vi "HFRR ADV v01.vi"() -> ()   [LabVIEW 2025] (continued)
          }
          frame #1 {
            n783 = local write "Tab Control 4"(T14."Air Step 3" ("Tab Control 4")) -> ()
          }
        }
      }
      event "Temperature Continue Step 3": Value Change {
        n784 = event-data() -> ()  [unwired: 1 in, 6 out]
        n785 = stacked-sequence {
          frame #0 {
            n786 = stacked-sequence {
              frame #0 {
                n787 = Wait (ms)(milliseconds to wait=u32 1500) -> ()  [unwired: 1 out]
              }
              frame #1 {
              }
              frame #2 {
              }
              frame #3 {
                # "CAL;A1;<true_T>"
                n788 = local write "Due Write"("CAL;A1;60" ("Command")) -> ()
              }
              frame #4 {
                n789 = Wait (ms)(milliseconds to wait=u32 1000) -> ()  [unwired: 1 out]
              }
              frame #5 {
                # "CAL;A1;<true_T>"
                n790 = local read "Sensor value"() -> (→"Sample 60deg temp":dbl)
                n791 = local write "Due Write"("CAL;A1;60" ("Command")) -> ()
              }
            }
          }
          frame #1 {
            w832 = 0.0
            w833 = 60.0
            n792 = local read "Sample 0deg temp"() -> (w843:dbl)
            n793 = local read "Sample 60deg temp"() -> (w842:dbl)
            n794 = Add(x=w833, y="Temperature diff") -> (x+y=w840:dbl)
            n795 = Subtract(x=w833, y="Temperature diff") -> (x-y=w839:dbl)
            n796 = Add(x=w832, y="Temperature diff") -> (x+y=w838:dbl)
            n797 = Subtract(x=w832, y="Temperature diff") -> (x-y=w837:dbl)
            n798 = In Range and Coerce(upper limit=w840, x=w842, lower limit=w839) -> (In Range?=w836:bool)  [unwired: 1 out]
            n799 = In Range and Coerce(upper limit=w838, x=w843, lower limit=w837) -> (In Range?=w835:bool)  [unwired: 1 out]
            n800 = And(x=w836, y=w835) -> (x .and. y?=w834:bool)
            n801 = case shown="True" w834 {
              frame False {
                n802 = property on="Accept & Save sample Temperature step 4" class="Bool (strict)"("DisabledEnum"=T20."Disabled" ("Disabled")) -> ()  [unwired: 2 in, 2 out]
                n803 = local write "Sample Temperature Calibration"(enum32{"True", "Fail"}."Fail" ("Sample Temperature Calibration  2")) -> ()
              }
              frame True {
                n804 = property on="Accept & Save sample Temperature step 4" class="Bool (strict)"("DisabledEnum"=T20."Enabled" ("Disabled")) -> ()  [unwired: 2 in, 2 out]
                n805 = local write "Sample Temperature Calibration"(enum32{"True", "Fail"}."True" ("Sample Temperature Calibration  2")) -> ()
              }
            }
          }
          frame #2 {
          }
          frame #3 {
          }
          frame #4 {
          }
          frame #5 {
          }
          frame #6 {
            # "CAL;END"
          }
          frame #7 {
          }
          frame #8 {
            # "CAL;END"
          }
          frame #9 {
            n806 = local write "Tab Control 4"(T14."Step 4" ("Tab Control 4")) -> ()
          }
        }
      }
      event "Accept & Save sample Temperature step 4": Value Change {
        n807 = event-data() -> ()  [unwired: 1 in, 6 out]
        n808 = stacked-sequence {
          frame #0 {
            n809 = local write "Due Write"("CAL;SAVE" ("Command")) -> ()
          }
          frame #1 {
            n810 = Wait (ms)(milliseconds to wait=u32 1000) -> ()  [unwired: 1 out]
          }
          frame #2 {
            n811 = local write "Due Write"("CAL;SAVE" ("Command")) -> ()
          }
          frame #3 {
            n812 = Wait (ms)(milliseconds to wait=u32 1000) -> ()  [unwired: 1 out]
          }
          frame #4 {
            n813 = local write "Due Write"("CAL;END" ("Command")) -> ()
          }
          frame #5 {
            n814 = Wait (ms)(milliseconds to wait=u32 1000) -> ()  [unwired: 1 out]
          }
          frame #6 {
            n815 = local write "Due Write"("CAL;END" ("Command")) -> ()
            n816 = local write "Temperature Selection"(T15."Default" ("Temperature Selection")) -> ()
            n817 = local write "Calibration Selection"(T10."Default" ("Calibration Selection")) -> ()
            n818 = local write "Tab Control 4"(T14."Main" ("Tab Control 4")) -> ()
            n819 = local write "Main Calibration Tab"(T9."Temperature" ("Main Calibration Tab")) -> ()
          }
          frame #7 {
            n820 = Get Date/Time In Seconds() -> (seconds since 1Jan1904=w862:timestamp)
            n821 = Format Into String(format string="%<%m/%d/%Y %I:%M:%S %p>T", w862) -> (resulting string=w860:string)  [unwired: 2 in, 1 out]
            n822 = local write "TEMPERATURE CALIBRATION"(w860) -> ()
          }
          frame #8 {
            n823 = local write "Save Button"(TRUE ("Save Button")) -> ()
            n824 = local write "Tab Control 4"(T14."Main" ("Tab Control 4")) -> ()
          }
        }
      }
      event "Accept & Save Air Temperature step 4": Value Change {
        n825 = event-data() -> ()  [unwired: 1 in, 6 out]
        n826 = stacked-sequence {
          frame #0 {
            n827 = local write "Due Write"("CAL;SAVE" ("Command")) -> ()
          }
          frame #1 {
            n828 = Wait (ms)(milliseconds to wait=u32 1000) -> ()  [unwired: 1 out]
          }
          frame #2 {
            n829 = local write "Due Write"("CAL;SAVE" ("Command")) -> ()
          }
          frame #3 {
            n830 = Wait (ms)(milliseconds to wait=u32 1000) -> ()  [unwired: 1 out]
          }
          frame #4 {
            n831 = local write "Due Write"("CAL;END" ("Command")) -> ()
          }
          frame #5 {
            n832 = Wait (ms)(milliseconds to wait=u32 1000) -> ()  [unwired: 1 out]
          }
          frame #6 {
            n833 = local write "Due Write"("CAL;END" ("Command")) -> ()
            n834 = local write "Tab Control 4"(T14."Main" ("Tab Control 4")) -> ()
            n835 = local write "Main Calibration Tab"(T9."Temperature" ("Main Calibration Tab")) -> ()
            n836 = local write "Temperature Selection"(T15."Default" ("Temperature Selection")) -> ()
            n837 = local write "Calibration Selection"(T10."Default" ("Calibration Selection")) -> ()
          }
          frame #7 {
            n838 = Get Date/Time In Seconds() -> (seconds since 1Jan1904=w878:timestamp)
            n839 = Format Into String(format string="%<%m/%d/%Y %I:%M:%S %p>T", w878) -> (resulting string=w877:string)  [unwired: 2 in, 1 out]
            n840 = local write "TEMPERATURE CALIBRATION"(w877) -> ()
          }
          frame #8 {
            n841 = local write "Tab Control 4"(T14."Main" ("Tab Control 4")) -> ()
            n842 = local write "Save Button"(TRUE ("Save Button")) -> ()
          }
        }
      }
      event "Temperature Continue Step 6": Value Change {
        n843 = event-data() -> ()  [unwired: 1 in, 6 out]
        n844 = stacked-sequence {
          frame #0 {
            n845 = stacked-sequence {
              frame #0 {
                n846 = Wait (ms)(milliseconds to wait=u32 1000) -> ()  [unwired: 1 out]
              }
              frame #1 {
              }
              frame #2 {
              }
              frame #3 {
                # "CAL;A1;<true_T>"
                n847 = local write "Due Write"("CAL;A1;60" ("Command")) -> ()
              }
              frame #4 {
                n848 = Wait (ms)(milliseconds to wait=u32 1000) -> ()  [unwired: 1 out]
              }
              frame #5 {
                # "CAL;A1;<true_T>"
                n849 = local write "Due Write"("CAL;A1;60" ("Command")) -> ()
              }
            }
          }
          frame #1 {
            n850 = local read "Sensor value"() -> (→"Air 60deg temp":dbl)
          }
          frame #2 {
          }
          frame #3 {
          }
          frame #4 {
          }
          frame #5 {
          }
          frame #6 {
            # "CAL;END"
          }
          frame #7 {
            w886 = 0.0 ("x")
            w887 = 60.0 ("x")
            n851 = local read "Temperature diff"() -> (w890:dbl)
            n852 = local read "Air 60deg temp"() -> (w889:dbl)
            n853 = local read "Air 0deg temp"() -> (w888:dbl)
            n854 = Add(x=w887, y=w890) -> (x+y=w897:dbl)
            n855 = Subtract(x=w887, y=w890) -> (x-y=w896:dbl)
            n856 = Add(x=w886, y=w890) -> (x+y=w895:dbl)
            n857 = Subtract(x=w886, y=w890) -> (x-y=w894:dbl)
            n858 = In Range and Coerce(upper limit=w897, x=w889, lower limit=w896) -> (In Range?=w893:bool)  [unwired: 1 out]
            n859 = In Range and Coerce(upper limit=w895, x=w888, lower limit=w894) -> (In Range?=w892:bool)  [unwired: 1 out]
            n860 = And(x=w893, y=w892) -> (x .and. y?=w891:bool)
            n861 = case shown="True" w891 {
              frame False {
                n862 = property on="Accept & Save Air Temperature step 4" class="Bool (strict)"("DisabledEnum"=T20."Disabled" ("Disabled")) -> ()  [unwired: 2 in, 2 out]
                n863 = local write "Air Temperature Calibration"(enum32{"True", "Fail"}."Fail" ("Sample Temperature Calibration  2")) -> ()
              }
              frame True {
                n864 = local write "Air Temperature Calibration"(enum32{"True", "Fail"}."True" ("Sample Temperature Calibration  2")) -> ()
                n865 = property on="Accept & Save Air Temperature step 4" class="Bool (strict)"("DisabledEnum"=T20."Enabled" ("Disabled")) -> ()  [unwired: 2 in, 2 out]
              }
            }
          }
          frame #8 {
            # "CAL;END"
          }
          frame #9 {
            n866 = local write "Tab Control 4"(T14."Air Step 4" ("Tab Control 4")) -> ()
          }
        }
      }
      event "Back Stroke step main temperature": Value Change {
        n867 = event-data() -> ()  [unwired: 1 in, 6 out]
        n868 = stacked-sequence {
          frame #0 {
            n869 = Wait (ms)(milliseconds to wait=u32 1000) -> ()  [unwired: 1 out]
          }
          frame #1 {
            # "CAL;END"
            n870 = local write "Due Write"("CAL;END" ("Command")) -> ()
          }
          frame #2 {
            n871 = Wait (ms)(milliseconds to wait=u32 1000) -> ()  [unwired: 1 out]
          }
          frame #3 {
            # "CAL;END"
            n872 = local write "Due Write"("CAL;END" ("Command")) -> ()
          }
          frame #4 {
            n873 = local write "Temperature Selection"(T15."Default" ("Temperature Selection")) -> ()
            n874 = local write "Calibration Selection"(T10."Default" ("Calibration Selection")) -> ()
            n875 = local write "Main Calibration Tab"(T9."Main" ("Main Calibration Tab")) -> ()
            n876 = local write "Tab Control 4"(T14."Main" ("Tab Control 4")) -> ()
          }
        }
      }
      event "TEMPERATURE STEP  Back 4", "TEMPERATURE STEP 1 Back 3", "TEMPERATURE STEP  Back 3", "TEMPERATURE STEP 1 Back 2", "Back Air TEMPERATURE Step 4", "Back SAMPLE TEMPERATURE Step 4": Value Change {
        # "Back Stroke step main temperature"
        n877 = event-data() -> ()  [unwired: 1 in, 6 out]
        n878 = stacked-sequence {
          frame #0 {
            n879 = Wait (ms)(milliseconds to wait=u32 1000) -> ()  [unwired: 1 out]
          }
          frame #1 {
            # "CAL;END"
            n880 = local write "Due Write"("CAL;END" ("Command")) -> ()
          }
          frame #2 {
            n881 = Wait (ms)(milliseconds to wait=u32 1000) -> ()  [unwired: 1 out]
          }
          frame #3 {
            # "CAL;END"
            n882 = local write "Due Write"("CAL;END" ("Command")) -> ()
          }
          frame #4 {
            # "TEMPERATURE STEP  Back 4"
            n883 = local write "Main Calibration Tab"(T9."Temperature" ("Main Calibration Tab")) -> ()
            n884 = local write "Temperature Selection"(T15."Default" ("Temperature Selection")) -> ()
            n885 = local write "Tab Control 4"(T14."Main" ("Tab Control 4")) -> ()
            n886 = local write "Calibration Selection"(T10."Default" ("Calibration Selection")) -> ()
          }
        }
      }
      event "FF BACK", "FF BACK 2", "FF BACK 3", "FF BACK 4", "FF BACK 5", "FF BACK 6": Value Change {
        n887 = event-data() -> ()  [unwired: 1 in, 6 out]
        n888 = stacked-sequence {
          frame #0 {
            n889 = Wait (ms)(milliseconds to wait=u32 1000) -> ()  [unwired: 1 out]
          }
          frame #1 {
            n890 = local write "Due Write"("VC;0") -> ()
          }
          frame #2 {
            n891 = Wait (ms)(milliseconds to wait=u32 1000) -> ()  [unwired: 1 out]
          }
          frame #3 {
            n892 = local write "Due Write"("VC;0") -> ()
          }
          frame #4 {
            w923 = FALSE
            n893 = local write "FF BACK 2"(w923) -> ()
            n894 = local write "FF BACK 3"(w923) -> ()
            n895 = local write "FF BACK 4"(w923) -> ()
            n896 = local write "FF BACK 5"(w923) -> ()
            n897 = local write "FF BACK 6"(w923) -> ()
            n898 = local write "FF BACK"(w923) -> ()
          }
          frame #5 {
            n899 = local write "Temperature Selection"(T15."Default" ("Temperature Selection")) -> ()
            n900 = local write "Calibration Selection"(T10."Default" ("Calibration Selection")) -> ()
            n901 = local write "Friction Force Tab"(T13."Page 1" ("Friction Force Tab")) -> ()
            n902 = local write "Main Calibration Tab"(T9."Main" ("Main Calibration Tab")) -> ()
            n903 = property on="Tab Control 6" class="TabCtl (strict)"("Visible"=FALSE) -> ()  [unwired: 2 in, 2 out]
            n904 = property on="Friction Force Calibration Result Tab" class="TabCtl (strict)"("Visible"=FALSE) -> ()  [unwired: 2 in, 2 out]
          }
        }
      }
      event "Accept & Save FF": Value Change {
        n905 = event-data() -> ()  [unwired: 1 in, 6 out]
        n906 = stacked-sequence {
          frame #0 {
            n907 = Wait (ms)(milliseconds to wait=u32 1000) -> ()  [unwired: 1 out]
          }
          frame #1 {
            n908 = local write "Due Write"("VC;0") -> ()
          }
          frame #2 {
            n909 = Wait (ms)(milliseconds to wait=u32 1000) -> ()  [unwired: 1 out]
          }
          frame #3 {
            n910 = local write "Due Write"("VC;0") -> ()
          }
          frame #4 {
            w934 = FALSE
            n911 = local write "FF BACK 2"(w934) -> ()
            n912 = local write "FF BACK 3"(w934) -> ()
            n913 = local write "FF BACK 4"(w934) -> ()
            n914 = local write "FF BACK 5"(w934) -> ()
            n915 = local write "FF BACK 6"(w934) -> ()
            n916 = local write "FF BACK"(w934) -> ()
          }
          frame #5 {
            n917 = Get Date/Time In Seconds() -> (seconds since 1Jan1904=w937:timestamp)
            n918 = Format Into String(format string="%<%m/%d/%Y %I:%M:%S %p>T", w937) -> (resulting string=w935:string)  [unwired: 2 in, 1 out]
            n919 = local write "FRICTION CALIBRATION"(w935) -> ()
          }
          frame #6 {
            n920 = local write "Temperature Selection"(T15."Default" ("Temperature Selection")) -> ()
            n921 = local write "Calibration Selection"(T10."Default" ("Calibration Selection")) -> ()
            n922 = local write "Friction Force Tab"(T13."Page 1" ("Friction Force Tab")) -> ()
            n923 = local write "Main Calibration Tab"(T9."Main" ("Main Calibration Tab")) -> ()
            n924 = local write "Save Button"(TRUE ("Save Button")) -> ()
            n925 = property on="Tab Control 6" class="TabCtl (strict)"("Visible"=FALSE) -> ()  [unwired: 2 in, 2 out]
            n926 = property on="Friction Force Calibration Result Tab" class="TabCtl (strict)"("Visible"=FALSE) -> ()  [unwired: 2 in, 2 out]
          }
        }
      }
      event "FF CONTINUE": Value Change {
        n927 = event-data() -> ()  [unwired: 1 in, 6 out]
        n928 = local write "FF CONTINUE"(FALSE ("FF CONTINUE")) -> ()
        n929 = local write "Friction Force Tab"(T13."Page 2" ("Friction Force Tab")) -> ()
      }
      event "FF CONTINUE 2": Value Change {
        n930 = event-data() -> ()  [unwired: 1 in, 6 out]
        n931 = local write "FF CONTINUE 2"(FALSE ("FF CONTINUE")) -> ()
        n932 = local write "Friction Force Tab"(T13."Page 3" ("Friction Force Tab")) -> ()
      }
      event "FF CONTINUE 3": Value Change {
        n933 = event-data() -> ()  [unwired: 1 in, 6 out]
        n934 = local write "FF CONTINUE 3"(FALSE ("FF CONTINUE")) -> ()
        n935 = local write "Friction Force Tab"(T13."Page 4" ("Friction Force Tab")) -> ()
      }
      event "FF CONTINUE 4": Value Change {
        n936 = event-data() -> ()  [unwired: 1 in, 6 out]
        n937 = local write "FF CONTINUE 4"(FALSE ("FF CONTINUE")) -> ()
        n938 = local write "Friction Force Tab"(T13."Page 5" ("Friction Force Tab")) -> ()
        n939 = property on="Friction Force Calibration Result Tab" class="TabCtl (strict)"("Visible"=FALSE) -> ()  [unwired: 2 in, 2 out]
      }
      event "FF CONTINUE 5": Value Change {
        n940 = event-data() -> ()  [unwired: 1 in, 6 out]
        n941 = local write "FF CONTINUE 5"(FALSE ("FF CONTINUE")) -> ()
        n942 = local write "Friction Force Tab"(T13."Page 6" ("Friction Force Tab")) -> ()
        n943 = property on="Friction Force Calibration Result Tab" class="TabCtl (strict)"("Visible"=FALSE) -> ()  [unwired: 2 in, 2 out]
        n944 = property on="Tab Control 6" class="TabCtl (strict)"("Visible"=FALSE) -> ()  [unwired: 2 in, 2 out]
      }
      event "Stroke Report Button": Value Change {
        n945 = event-data() -> ()  [unwired: 1 in, 6 out]
        n946 = local read "Point 5 - 1.0 mm"() -> (w959:bool)
        n947 = case shown="False" w959 {
          tunnel: [0.8 1.0] -> w958
          frame False {
          }
          frame True {
          }
        }
        n948 = local read "Machine Serial Number"() -> (w962:string)
        n949 = local read "USERNAME"() -> (w960:string)
        n950 = local write "Stroke Report Button"(FALSE ("Stroke Report Button")) -> ()
        n951 = call "Stroke Calibration Report.vi"("measured_value"=w958, "operator_name"=w960, "Instrument_serial Number"=w962) -> ()  [unwired: 7 in, 2 out]
      }
      event "Sample Report Button": Value Change {
        n952 = event-data() -> ()  [unwired: 1 in, 6 out]
        n953 = local read "Machine Serial Number"() -> (w968:string)
        n954 = local read "Sample 0deg temp"() -> (w965:dbl)
        n955 = local read "Sample 60deg temp"() -> (w966:dbl)
        n956 = local read "USERNAME"() -> (w967:string)
        n957 = call "Temperature Calibration Report.vi"("measured_60"=w966, "measured_zero"=w965, "operator_name"=w967, "Instrument_serial Number"=w968) -> ()  [unwired: 6 in, 2 out]
        n958 = local write "Sample Report Button"(FALSE ("Sample Report Button")) -> ()
      }
      event "Report Button FF": Value Change {
        n959 = event-data() -> ()  [unwired: 1 in, 6 out]
        n960 = local read "FF PASS"() -> (w973:bool)
        n961 = local read "Machine Serial Number"() -> (w976:string)
        n962 = Select(t="PASS", s=w973, f="FAIL") -> (s? t:f=w970:string)
        n963 = local read "USERNAME"() -> (w975:string)
        n964 = call "FF Calibration Report.vi"("pass_or_fail"=w970, "operator_name"=w975, "Instrument_serial Number"=w976) -> ()  [unwired: 7 in, 2 out]
        n965 = local write "Report Button FF"(FALSE ("Sample Report Button")) -> ()
      }
      event "Air Temperature Report Button": Value Change {
        n966 = event-data() -> ()  [unwired: 1 in, 6 out]
        n967 = local read "Machine Serial Number"() -> (w981:string)
        n968 = local read "Air 0deg temp"() -> (w978:dbl)
        n969 = local read "Air 60deg temp"() -> (w979:dbl)
        n970 = local read "USERNAME"() -> (w980:string)
        n971 = call "Air Temperature Calibration Report.vi"("measured_60"=w979, "measured_zero"=w978, "operator_name"=w980, "Instrument_serial Number"=w981) -> ()  [unwired: 6 in, 2 out]
        n972 = local write "Air Temperature Report Button"(FALSE ("Sample Report Button")) -> ()
      }
      event "Quit": Value Change {
        n973 = event-data() -> ()  [unwired: 1 in, 6 out]
      }
    }
    n974 = Wait (ms)(milliseconds to wait=u32 100) -> ()  [unwired: 1 out]
  }
  n975 = while {
    shift-right: [w984] -> _
    shift-left: "Enum - Selector" -> [w985]
    stop <- w986 stop-if-true
    # "Auto Start Logic Loop"
    n976 = case shown="\"close\"" w985 {
      tunnel: [w989 w995 w1023 w1058 w1088 Auto_Start_enum."Exit" ("Enum - Selector") Auto_Start_enum."Init" ("Enum - Selector")] -> w984
      frame "Init", Default {
        n977 = local read "Auto Start Test"() -> (w988:bool)
        n978 = Select(t=Auto_Start_enum."Humidity & Temperature On" ("Enum - Selector"), s=w988, f=Auto_Start_enum."Init") -> (s? t:f=w989:T17)
      }
      frame "Humidity & Temperature On" {
        n979 = stacked-sequence {
          tunnel: [_ _ _ _ _ _ Auto_Start_enum."Reach point" ("Enum - Selector")] -> w992
          frame #0 {
            w997 = T20."Disabled and Grayed Out" ("Disabled")
            w998 = TRUE ("Heater Button")
            n980 = property on="Humidity" class="Bool (strict)"("DisabledEnum"=w997) -> ()  [unwired: 2 in, 2 out]
            n981 = property on="Heater Button" class="Bool (strict)"("DisabledEnum"=w997) -> ()  [unwired: 2 in, 2 out]
            n982 = local write "Heater Button"(w998) -> ()
            n983 = local write "Humidity"(w998) -> ()
            n984 = property on="Heater Button" class="Bool (strict)"("Val(Sgnl)"=TRUE ("Value (Signaling)")) -> ()  [unwired: 2 in, 2 out]
          }
          frame #1 {
            n985 = Wait (ms)(milliseconds to wait=u32 3000) -> ()  [unwired: 1 out]
          }
          frame #2 {
            n986 = local read "Set Temp"() -> (w1004:dbl)
            n987 = Number To Fractional String(number=w1004, precision (6)=i16 2) -> (F-format string=w1001:string)  [unwired: 2 in]
            n988 = Concatenate Strings("ST;" ("Command"), w1001) -> (w1002:string)
            n989 = local write "Due Write"(w1002) -> ()
          }
          frame #3 {
            n990 = Wait (ms)(milliseconds to wait=u32 1500) -> ()  [unwired: 1 out]
          }
          frame #4 {
            (unwired) i16 2 ("precision (6)")
            n991 = local read "WriteHumidity"() -> (w1006:string[])
            n992 = local read "Set Rh"() -> (w1009:dbl)
            n993 = Number To Fractional String(number=w1009) -> (F-format string=w1010:string)  [unwired: 3 in]
            n994 = Concatenate Strings("M;" ("new element/subarray"), w1010) -> (w1011:string)
            n995 = Insert Into Array(array=w1006, new element=w1011) -> (w1007:string[])  [unwired: 1 in]
            n996 = local write "WriteHumidity"(w1007) -> ()
            n997 = local write "Due Write"("HE;1" ("Command")) -> ()
          }
          frame #5 {
            n998 = Wait (ms)(milliseconds to wait=u32 1500) -> ()  [unwired: 1 out]
          }
          frame #6 {
            w1014 = TRUE ("Reach point temp")
            n999 = local write "Reach point Humidity"(w1014) -> ()
            n1000 = local write "Reach point temp"(w1014) -> ()
          }
        }
        n1001 = local read "Auto Start Test"() -> (w994:bool)
        n1002 = Not(x=w994) -> (.not. x?=w993:bool)
        n1003 = Select(t=Auto_Start_enum."close", s=w993, f=w992) -> (s? t:f=w995:T17)
      }
      frame "Reach point" {
        w1024 = TRUE ("PAUSE")
        w1032 = 1.0 ("y")
        w1035 = 1.0 ("y")
        n1004 = local read "Set Temp"() -> (w1017:dbl)
        n1005 = local read "Set Humidity:"() -> (w1031:dbl)
        n1006 = local read "Humidity ( %RH )"() -> (w1036:dbl)
        n1007 = Add(x=w1017, y=w1035) -> (x+y=w1034:dbl)
        n1008 = Subtract(x=w1017, y=w1035) -> (x-y=w1033:dbl)
        n1009 = Add(x=w1031, y=w1032) -> (x+y=w1030:dbl)
        n1010 = Subtract(x=w1031, y=w1032) -> (x-y=w1029:dbl)
        n1011 = local read "TEMP"() -> (w1037:dbl)
        n1012 = In Range and Coerce(upper limit=w1030, x=w1036, lower limit=w1029) -> (In Range?=w1018:bool)  [unwired: 1 out]
        n1013 = In Range and Coerce(upper limit=w1034, x=w1037, lower limit=w1033) -> (In Range?=w1019:bool)  [unwired: 1 out]
        n1014 = disable-structure shown="Enabled" {
          disable-tunnel: w1018 -> [w1038 _]
          disable-tunnel: [w1038 TRUE] -> w1016
          frame Disabled {
            n1015 = case shown="True" w1038 {
              frame False {
              }
              frame True {
                n1016 = case shown="True" "Reach point Humidity" {
                  selector: "Reach point Humidity" -> [_ w1044]
                  frame False {
                  }
                  frame True {
                    n1017 = local read "EVENT LOG"() -> (w1041:string)
                    n1018 = Not(x=w1044) -> (.not. x?=w1043:bool)
                    n1019 = local write "Reach point Humidity"(w1043) -> ()
                    n1020 = call "Event Log.vi"("Content"="Target Humidity reached", "EVENT LOG"=w1041) -> ("EVENT LOG"=w1042:string)  [unwired: 8 in, 1 out]
                    n1021 = local write "EVENT LOG"(w1042) -> ()
                  }
                }
              }
            }
          }
          frame Enabled {
          }
        }
        n1022 = case shown="True" w1019 {
          frame False {
          }
          frame True {
            n1023 = case shown="True" "Reach point temp" {
              selector: "Reach point temp" -> [_ w1051]
              frame False {
              }
              frame True {
                n1024 = local read "EVENT LOG"() -> (w1048:string)
                n1025 = Not(x=w1051) -> (.not. x?=w1050:bool)
                n1026 = local write "Reach point temp"(w1050) -> ()
                n1027 = call "Event Log.vi"("Content"="Target Temperature reached", "EVENT LOG"=w1048) -> ("EVENT LOG"=w1049:string)  [unwired: 8 in, 1 out]
                n1028 = local write "EVENT LOG"(w1049) -> ()
              }
            }
          }
        }
        n1029 = local read "Auto Start Test"() -> (w1022:bool)
        n1030 = And(x=w1019, y=w1016) -> (x .and. y?=w1028:bool)
        n1031 = Select(t=Auto_Start_enum."Maintain Stage" ("Enum - Selector"), s=w1028, f=Auto_Start_enum."Reach point" ("Enum - Selector")) -> (s? t:f=w1025:T17)
        n1032 = Not(x=w1022) -> (.not. x?=w1021:bool)
        n1033 = Select(t=Auto_Start_enum."close", s=w1021, f=w1025) -> (s? t:f=w1023:T17)
        n1034 = call "ELAPSED TIMER VI.vi"("RESET"=w1024, "PAUSE"=w1024) -> ()  [unwired: 7 in, 3 out]
      }
      frame "Maintain Stage" {
        w1066 = 2.0 ("y")
        w1065 = 1.0 ("y")
        # "Humidity and temperature set point has stabilized."
        # "Humidity and  temperatures Set Point  have been reached"
        n1035 = local read "Set Temp"() -> (w1053:dbl)
        n1036 = local read "Set Humidity:"() -> (w1069:dbl)
        n1037 = local read "Humidity ( %RH )"() -> (w1072:dbl)
        n1038 = Add(x=w1053, y=w1065) -> (x+y=w1071:dbl)
        n1039 = Subtract(x=w1053, y=w1065) -> (x-y=w1070:dbl)
        n1040 = local read "TEMP"() -> (w1073:dbl)
        n1041 = Add(x=w1069, y=w1066) -> (x+y=w1068:dbl)
        n1042 = Subtract(x=w1069, y=w1066) -> (x-y=w1067:dbl)
        n1043 = In Range and Coerce(upper limit=w1071, x=w1073, lower limit=w1070) -> (In Range?=w1064:bool)  [unwired: 1 out]
        n1044 = In Range and Coerce(upper limit=w1068, x=w1072, lower limit=w1067) -> ()  [unwired: 2 out]
        n1045 = And(x=w1064, y=TRUE) -> (x .and. y?=w1063:bool)
        n1046 = Not(x=w1063) -> (.not. x?=w1062:bool)
        n1047 = call "ELAPSED TIMER VI.vi"("TARGET"=60.0, "RESET"=w1062, "PAUSE"=FALSE) -> ("ELAPSED INDICATION"=w1059:bool)  [unwired: 6 in, 2 out]
        n1048 = case shown="True" w1059 {
          tunnel: w1059 -> [_ w1076]
          tunnel: [Auto_Start_enum."Maintain Stage" ("Enum - Selector") w1075] -> w1057
          frame False {
          }
          frame True {
            n1049 = stacked-sequence {
              tunnel: w1076 -> [_ _ _ _ _]
              tunnel: [_ _ _ _ Auto_Start_enum."Start Stage" ("Enum - Selector")] -> w1075
              frame #0 {
                n1050 = local read "EVENT LOG"() -> (w1078:string)
                n1051 = call "Event Log.vi"("Content"="Temperature set point has stabilized.", "EVENT LOG"=w1078) -> ("EVENT LOG"=w1079:string)  [unwired: 8 in, 1 out]
                n1052 = local write "EVENT LOG"(w1079) -> ()
              }
              frame #1 {
                n1053 = Wait (ms)(milliseconds to wait=u32 100) -> ()  [unwired: 1 out]
              }
              frame #2 {
                n1054 = local read "EVENT LOG"() -> (w1083:string)
                n1055 = call "Event Log.vi"("Content"="Auto Test Started", "EVENT LOG"=w1083) -> ("EVENT LOG"=w1084:string)  [unwired: 8 in, 1 out]
                n1056 = local write "EVENT LOG"(w1084) -> ()
                n1057 = local write "FRICVALZ 4"(TRUE ("FRICVALZ 4")) -> ()
              }
              frame #3 {
                w1085 = TRUE ("RUN")
                n1058 = local write "RUN"(w1085) -> ()
                n1059 = property on="Auto Start Temp" class="Bool (strict)"("Val(Sgnl)"=w1085) -> ()  [unwired: 2 in, 2 out]
                "Auto Start Temp" <- w1085
              }
              frame #4 {
              }
            }
          }
        }
        n1060 = local read "Auto Start Test"() -> (w1056:bool)
        n1061 = Not(x=w1056) -> (.not. x?=w1055:bool)
        n1062 = Select(t=Auto_Start_enum."close", s=w1055, f=w1057) -> (s? t:f=w1058:T17)
      }
      frame "Start Stage" {
        w1087 = TRUE ("PAUSE")
        n1063 = local read "Auto Start Test"() -> (w1092:bool)
        n1064 = Not(x=w1092) -> (.not. x?=w1091:bool)
        n1065 = Select(t=Auto_Start_enum."close" ("Enum - Selector"), s=w1091, f=Auto_Start_enum."Start Stage" ("Enum - Selector")) -> (s? t:f=w1088:T17)
        n1066 = call "ELAPSED TIMER VI.vi"("RESET"=w1087, "PAUSE"=w1087) -> ()  [unwired: 7 in, 3 out]
      }
      frame "close" {
        w1095 = FALSE ("Heater Button")
        n1067 = local write "RUN"(w1095) -> ()
        n1068 = local write "Heater Button"(w1095) -> ()
        n1069 = local write "Humidity"(w1095) -> ()
        n1070 = local write "Auto Start Test"(w1095) -> ()
        n1071 = property on="Heater Button" class="Bool (strict)"("Val(Sgnl)"=FALSE ("Value (Signaling)")) -> ()  [unwired: 2 in, 2 out]
        n1072 = local write "Humidity 2"(TRUE ("Humidity")) -> ()
      }
      frame "Exit" {
      }
    }
    n1073 = Wait (ms)(milliseconds to wait=u32 100) -> ()  [unwired: 1 out]
    n1074 = local read "Quit"() -> (w986:bool)
  }
  n1075 = property on="Service Password Log" class="Str"("Visible"=w27) -> ()  [unwired: 2 in, 2 out]
  n1076 = property on="Password 3" class="Clust (strict)"("Visible"=w27) -> ()  [unwired: 2 in, 2 out]
  n1077 = while {
    stop <- w1124 stop-if-true
    w1107 = errorcluster {"status"=FALSE, "code"=0, "source"=""} ("error in (no error) 3")
    # "this loop is for manual report generation"
    n1078 = local read "Confirm Measrurement"() -> (w1106:bool)
    n1079 = case shown="True" w1106 {
      selector: w1106 -> [_ w1214]
      tunnel: errorcluster {"status"=FALSE, "code"=0, "source"=""} ("error in (no error) 3") -> [_ w1215]
      tunnel: [_ w1213] -> _
      frame False {
      }
      frame True {
        n1080 = stacked-sequence {
          tunnel: w1215 -> [_ w1248 _]
          tunnel: w1214 -> [_ _ w1355]
          tunnel: [_ w1236 _] -> w1213
          frame #0 {
            n1081 = String To Path(string="C:\\LAB-IQ\\Image Calibrate v01.dcf") -> (path=w1218:path)
            n1082 = Open/Create/Replace File ("Open File")(file path (use dialog)=w1218) -> (refnum out=w1219:refnum<file>)  [unwired: 5 in, 2 out]
            n1083 = for {
              N: 4 -> [_]
              tunnel: w1219 -> [w1225]
              i -> [w1221]
              n1084 = Read from Text File ("Read File")(file (use dialog)=w1225) -> (text=w1226:string)  [unwired: 3 in, 3 out]
              n1085 = String Subset(string=w1226, offset (0)=6, length (rest)=10 ("length (rest)")) -> (substring=w1222:string)
              n1086 = Fract/Exp String To Number(string=w1222) -> (number=w1220:dbl)  [unwired: 3 in, 1 out]
              n1087 = case shown="3" w1221 {
                tunnel: w1220 -> [w1227 w1228 _ w1229 _]
                frame 0 {
                  n1088 = local write "5x Gain"(w1227) -> ()
                }
                frame 1 {
                  n1089 = local write "10x Gain"(w1228) -> ()
                }
                frame 2 {
                }
                frame 3 {
                  n1090 = local write "100x gain"(w1229) -> ()
                }
                frame 4, Default {
                }
              }
            }
          }
          frame #1 {
            n1091 = local read "TEST STANDARD"() -> (w1231:T5)
            n1092 = case shown="\"ISO 12156\"" w1231 {
              tunnel: ["ASTM D6079" "ISO 12156"] -> w1230
              frame "ASTM D6079", Default {
              }
              frame "ISO 12156" {
              }
            }
            n1093 = call "IMAGE ANALYSIS.vi"("Enum"=POST_ANALYSIS_ENUM."GET MEASUREMENTS", "error in"=w1248) -> ("error out"=w1255:errorcluster)  [unwired: 8 in, 1 out]
            n1094 = local read "Magnification :"() -> (w1241:string)
            n1095 = call "Stall Data Flow.vim"("value in"=w1255, "milliseconds to wait"=u32 1000) -> ("value out"=w1254:errorcluster)  [unwired: 1 out]
            n1096 = local read "Test File List :"() -> (w1252:string)
            n1097 = case shown="\"10x\"" w1241 {
              tunnel: [w1291 w1292] -> w1239
              frame "5x", Default {
                n1098 = local read "5x Gain"() -> (w1291:dbl)
              }
              frame "10x" {
                # "5x"
                n1099 = local read "10x Gain"() -> (w1292:dbl)
              }
            }
            n1100 = call "IMAGE ANALYSIS.vi"("Enum"=POST_ANALYSIS_ENUM."READ", "error in"=w1254) -> ("error out"=w1251:errorcluster, "data out"=w1242:string)  [unwired: 8 in]
            n1101 = Match Pattern(string=w1242, regular expression="\"type\": ") -> (after substring=w1246:string)  [unwired: 1 in, 3 out]
            n1102 = call "IMAGE PATH CREATION PY.vi"("error in (no error)"=w1251, "File Name :"=w1252) -> ("error out"=w1250:errorcluster, "File Path"=w1238:path, "File Path String:"=w1233:string)  [unwired: 7 in]
            n1103 = Match Pattern(string=w1246, regular expression=",") -> (before substring=w1232:string)  [unwired: 1 in, 3 out]
            n1104 = local read "Calibration Tab"() -> (w1235:enum32{"Measrument", "Calibrate"})
            n1105 = call "Stall Data Flow.vim"("value in"=w1250, "milliseconds to wait"=u32 250) -> ("value out"=w1234:errorcluster)  [unwired: 1 out]
            n1106 = Equal?(x=w1232, y="\"rectangle\"") -> (x = y?=w1243:bool)
            n1107 = case shown="False" w1243 {
              tunnel: w1242 -> [w1297 w1352]
              tunnel: w1239 -> [_ w1343]
              tunnel: cluster{"major":dbl, "minor":dbl, "average":dbl} {"major"=0.0, "minor"=0.0, "average"=0.0} -> [w1295 w1339]
              tunnel: [w1294 w1336] -> w1237
              tunnel: w1232 -> [w1296 _]
              tunnel: w1239 -> [w1293 _]
              frame False {
                n1108 = Equal?(x=w1296, y="\"line\"") -> (x = y?=w1298:bool)
                n1109 = case shown="True" w1298 {
                  tunnel: w1297 -> [_ w1313]
                  tunnel: w1295 -> [w1300 w1312]
                  tunnel: [w1300 w1310] -> w1294
                  tunnel: w1293 -> [_ w1309]
                  frame False {
                  }
                  frame True {
                    w1308 = 0.0 ("Major Axis")
                    n1110 = Match Pattern(string=w1313, regular expression="\"length_px\":") -> (after substring=w1311:string)  [unwired: 1 in, 3 out]
                    n1111 = property on="Major Axis" class="DigNum (strict)"("Caption.Text"="") -> ()  [unwired: 2 in, 2 out]
                    n1112 = property on="Minor Axis" class="DigNum (strict)"("Caption.Text"="") -> ()  [unwired: 2 in, 2 out]
                    n1113 = property on="Average" class="DigNum (strict)"("Caption.Text"="Line") -> ()  [unwired: 2 in, 2 out]
                    n1114 = Fract/Exp String To Number(string=w1311, default (0 dbl)=0.0 ("default (0 DBL)")) -> (number=w1307:dbl)  [unwired: 2 in, 1 out]
                    "Pixel Value" <- w1307
                    n1115 = Multiply(x=w1307, y=w1309) -> (x*y=w1320:dbl)
                    n1116 = Multiply(x=w1320, y=1000.0) -> (x*y=w1303:dbl)
                    n1117 = Divide(x=w1303, y=1000.0) -> (x/y=w1306:dbl)
                    n1118 = local write "Measurment (mm)"(w1306) -> ()
                    n1119 = Bundle By Name(cluster=w1312, "average"=w1303) -> (w1310:cluster{"major":dbl, "minor":dbl, "average":dbl})
                    n1120 = Number To Fractional String(number=w1303, precision (6)=i16 1) -> (F-format string=w1302:string)  [unwired: 2 in]
                    n1121 = local write "Minor Axis"(w1308) -> ()
                    n1122 = local write "Major Axis"(w1308) -> ()
                    n1123 = Fract/Exp String To Number(string=w1302) -> (number=w1301:dbl)  [unwired: 3 in, 1 out]
                    n1124 = local write "Average"(w1301) -> ()
                  }
                }
              }
              frame True {
                w1340 = 1000.0 ("y")
                w1346 = 0.0 ("default (0 DBL)")
                n1125 = Match Pattern(string=w1352, regular expression=" \"width_px\":") -> (after substring=w1350:string)  [unwired: 1 in, 3 out]
                n1126 = Match Pattern(string=w1350, regular expression="\"height_px\":") -> (before substring=w1348:string, after substring=w1347:string)  [unwired: 1 in, 2 out]
                n1127 = Fract/Exp String To Number(string=w1348, default (0 dbl)=w1346) -> (number=w1345:dbl)  [unwired: 2 in, 1 out]
                n1128 = Fract/Exp String To Number(string=w1347, default (0 dbl)=w1346) -> (number=w1344:dbl)  [unwired: 2 in, 1 out]
                n1129 = Multiply(x=w1345, y=w1343) -> (x*y=w1342:dbl)
                n1130 = Multiply(x=w1344, y=w1343) -> (x*y=w1341:dbl)
                n1131 = Multiply(x=w1342, y=w1340) -> (x*y=w1326:dbl)
                n1132 = Multiply(x=w1341, y=w1340) -> (x*y=w1324:dbl)
                n1133 = Add(x=w1326, y=w1324) -> (x+y=w1338:dbl)
                n1134 = property on="Major Axis" class="DigNum (strict)"("Caption.Text"="Major Axis") -> ()  [unwired: 2 in, 2 out]
                n1135 = property on="Minor Axis" class="DigNum (strict)"("Caption.Text"="Minor Axis") -> ()  [unwired: 2 in, 2 out]
                n1136 = property on="Average" class="DigNum (strict)"("Caption.Text"="Average") -> ()  [unwired: 2 in, 2 out]
                n1137 = Divide(x=w1338, y=2.0) -> (x/y=w1322:dbl)
                n1138 = Bundle By Name(cluster=w1339, "major"=w1326, "minor"=w1324, "average"=w1322) -> (w1336:cluster{"major":dbl, "minor":dbl, "average":dbl})
                n1139 = Number To Fractional String(number=w1324, precision (6)=i16 1) -> (F-format string=w1331:string)  [unwired: 2 in]
                n1140 = Number To Fractional String(number=w1322, precision (6)=i16 1) -> (F-format string=w1332:string)  [unwired: 2 in]
                n1141 = Number To Fractional String(number=w1326, precision (6)=i16 1) -> (F-format string=w1330:string)  [unwired: 2 in]
                n1142 = Fract/Exp String To Number(string=w1331) -> (number=w1323:dbl)  [unwired: 3 in, 1 out]
                n1143 = Fract/Exp String To Number(string=w1332) -> (number=w1321:dbl)  [unwired: 3 in, 1 out]
                n1144 = Fract/Exp String To Number(string=w1330) -> (number=w1325:dbl)  [unwired: 3 in, 1 out]
                n1145 = local write "Major Axis"(w1325) -> ()
                n1146 = local write "Average"(w1321) -> ()
                n1147 = local write "Minor Axis"(w1323) -> ()
              }
            }
            n1148 = case shown="\"Measrument\", Default" w1235 {
              tunnel: w1238 -> [w1265 _]
              tunnel: w1237 -> [w1264 _]
              tunnel: [w1261 w1290] -> w1236
              tunnel: w1234 -> [w1263 w1290]
              tunnel: w1233 -> [w1262 _]
              tunnel: w1230 -> [w1260 _]
              frame "Measrument", Default {
                n1149 = stacked-sequence {
                  tunnel: w1265 -> [w1283 _]
                  tunnel: w1264 -> [w1281 _]
                  tunnel: w1263 -> [w1279 _]
                  tunnel: w1262 -> [w1278 _]
                  tunnel: [w1273 _] -> w1261
                  tunnel: w1260 -> [w1266 _]
                  frame #0 {
                    n1150 = call "IMAGE ANALYSIS.vi"("Enum"=POST_ANALYSIS_ENUM."SAVE IMAGE", "error in"=w1279, "IMAGE FILE PATH"=w1278) -> ("error out"=w1277:errorcluster)  [unwired: 7 in, 1 out]
                    n1151 = call "Stall Data Flow.vim"("value in"=w1277, "milliseconds to wait"=u32 1000) -> ("value out"=w1268:errorcluster)  [unwired: 1 out]
                    n1152 = local read "Test File List :"() -> (w1285:string)
                    n1153 = call "IMAGE ANALYSIS.vi"("Enum"=POST_ANALYSIS_ENUM."MINIMIZE UI", "error in"=w1268) -> ("error out"=w1275:errorcluster)  [unwired: 8 in, 1 out]
                    n1154 = Bundle By Name(cluster=T27 {"File Name"="", "Test Method"="", "Operator"="", "Fuel Description"="", "Date and time"=""} ("Main Ref"), "Test Method"=w1266, "File Name"=w1285) -> (w1286:T27)
                    n1155 = call "Stall Data Flow.vim"("value in"=w1275, "milliseconds to wait"=u32 1500) -> ("value out"=w1270:errorcluster)  [unwired: 1 out]
                    n1156 = call "duf file read.vi"("error in (no error)"=w1270, "Main Ref"=w1286) -> ("error out"=w1284:errorcluster, "Main Ref 2"=w1282:T27)  [unwired: 8 in]
                    n1157 = call "DETECTION REPORT for manual.vi"("error in (no error)"=w1284, "return value 3"=w1281, "Image File Path"=w1283, "Main Ref"=w1282) -> ("error out"=w1280:errorcluster)  [unwired: 7 in]
                    n1158 = call <vilib>:"Clear Errors.vi"("error in (no error)"=w1280) -> ("error out"=w1271:errorcluster)  [unwired: 5 in, 1 out]
                    n1159 = call "IMAGE ANALYSIS.vi"("Enum"=POST_ANALYSIS_ENUM."MINIMIZE UI", "error in"=w1271) -> ("error out"=w1273:errorcluster)  [unwired: 8 in, 1 out]
                  }
                  frame #1 {
                    n1160 = local write "Main Tab"(T4."HOME" ("Main Tab")) -> ()
                    n1161 = local write "Main Dashboard Buttons"(T1."Home" ("Main Dashboard Buttons")) -> ()
                  }
                }
              }
              frame "Calibrate" {
              }
            }
          }
          frame #2 {
            n1162 = Not(x=w1355) -> (.not. x?=w1354:bool)
            n1163 = local write "Confirm Measrurement"(w1354) -> ()
            n1164 = local read "Calibration Tab"() -> (w1353:enum32{"Measrument", "Calibrate"})
            n1165 = case shown="\"Measrument\", Default" w1353 {
              frame "Measrument", Default {
                (unwired) T22."HOME" ("Main Tab")
                n1166 = local write "Main Tab"(T4."HOME" ("Main Tab")) -> ()
              }
              frame "Calibrate" {
              }
            }
          }
        }
      }
    }
    n1167 = local read "Humidity"() -> (w1098:bool)
    n1168 = local read "Save Change"() -> (w1103:bool)
    n1169 = local read "Calibrate"() -> (w1104:bool)
    n1170 = local read "Auto Start Test"() -> (w1099:bool)
    n1171 = case shown="True" w1104 {
      selector: w1104 -> [_ w1211]
      frame False {
      }
      frame True {
        n1172 = Not(x=w1211) -> (.not. x?=w1210:bool)
        n1173 = local write "Calibrate"(w1210) -> ()
        n1174 = local write "Calibration Tab"(enum32{"Measrument", "Calibrate"}."Calibrate" ("Calibration Tab")) -> ()
      }
    }
    n1175 = case shown="True" w1103 {
      selector: w1103 -> [_ w1155]
      frame False {
      }
      frame True {
        n1176 = stacked-sequence {
          tunnel: w1155 -> [_ _ _ _ w1209]
          frame #0 {
            n1177 = call "IMAGE ANALYSIS.vi"("Enum"=POST_ANALYSIS_ENUM."HIDE UI") -> ()  [unwired: 9 in, 2 out]
          }
          frame #1 {
            n1178 = local read "100x gain"() -> (w1157:dbl)
            n1179 = local read "10x Gain"() -> (w1158:dbl)
            n1180 = local read "5x Gain"() -> (w1159:dbl)
            n1181 = Number To Fractional String(number=w1158, width (-)=i16 4, precision (6)=i16 7) -> (F-format string=w1180:string)  [unwired: 1 in]
            n1182 = Number To Fractional String(number=0.0, width (-)=i16 4, precision (6)=i16 7) -> (F-format string=w1175:string)  [unwired: 1 in]
            n1183 = Number To Fractional String(number=w1157, width (-)=i16 4, precision (6)=i16 7) -> (F-format string=w1163:string)  [unwired: 1 in]
            n1184 = Number To Fractional String(number=w1159, width (-)=i16 10 ("precision (6)"), precision (6)=i16 7) -> (F-format string=w1189:string)  [unwired: 1 in]
            n1185 = Concatenate Strings("[CH1]" ("string"), w1189, " - 5x Gain" ("string"), "\r") -> (w1179:string)
            n1186 = Concatenate Strings("[CH2]" ("string"), w1180, " - 10x Gain" ("string"), "\r") -> (w1178:string)
            n1187 = Concatenate Strings("[CH3]" ("string"), w1175, " - 20x Gain" ("string"), "\r") -> (w1169:string)
            n1188 = Concatenate Strings("[CH4]" ("string"), w1163, " - 100x Gain" ("string"), "\r") -> (w1162:string)
            n1189 = String To Path(string="C:\\LAB-IQ\\Image Calibrate v01.dcf") -> (path=w1192:path)
            n1190 = Concatenate Strings(w1179, w1178, w1169, w1162) -> (w1177:string)
            n1191 = call <vilib>:"Write Characters To File.vi"("append to file? (new file:F)"=FALSE, "character string"=w1177, "file path (dialog if empty)"=w1192) -> ()  [unwired: 2 in, 1 out]
          }
          frame #2 {
            n1192 = String To Path(string="C:\\LAB-IQ\\Image Calibrate v01.dcf") -> (path=w1195:path)
            n1193 = Open/Create/Replace File ("Open File")(file path (use dialog)=w1195) -> (refnum out=w1196:refnum<file>)  [unwired: 5 in, 2 out]
            n1194 = for {
              N: 4 -> [_]
              tunnel: w1196 -> [w1202]
              i -> [w1198]
              n1195 = Read from Text File ("Read File")(file (use dialog)=w1202) -> (text=w1203:string)  [unwired: 3 in, 3 out]
              n1196 = String Subset(string=w1203, offset (0)=6, length (rest)=10 ("length (rest)")) -> (substring=w1199:string)
              n1197 = Fract/Exp String To Number(string=w1199) -> (number=w1197:dbl)  [unwired: 3 in, 1 out]
              n1198 = case shown="3" w1198 {
                tunnel: w1197 -> [w1204 w1205 _ w1206 _]
                frame 0 {
                  n1199 = local write "5x Gain"(w1204) -> ()
                }
                frame 1 {
                  n1200 = local write "10x Gain"(w1205) -> ()
                }
                frame 2 {
                }
                frame 3 {
                  n1201 = local write "100x gain"(w1206) -> ()
                }
                frame 4, Default {
                }
              }
            }
          }
          frame #3 {
            n1202 = call "IMAGE ANALYSIS.vi"("Enum"=POST_ANALYSIS_ENUM."SHOW UI") -> ()  [unwired: 9 in, 2 out]
          }
          frame #4 {
            n1203 = Not(x=w1209) -> (.not. x?=w1208:bool)
            n1204 = local write "Save Change"(w1208) -> ()
          }
        }
      }
    }
    n1205 = case shown="False" w1099 {
      tunnel: w1098 -> [w1125 _]
      frame False {
        n1206 = case shown="True" w1125 {
          frame False {
          }
          frame True {
            n1207 = local read "Set Humidity:"() -> (w1129:dbl)
            n1208 = local read "Set Humidity:"() -> (w1132:dbl)
            n1209 = local read "Humidity ( %RH )"() -> (w1133:dbl)
            n1210 = Subtract(x=w1129, y=2.0) -> (x-y=w1127:dbl)
            n1211 = Add(x=w1132, y=2.0) -> (x+y=w1128:dbl)
            n1212 = In Range and Coerce(upper limit=w1128, x=w1133, lower limit=w1127) -> (In Range?=w1126:bool)  [unwired: 1 out]
            n1213 = case shown="True" w1126 {
              frame False {
              }
              frame True {
                n1214 = case shown="True" "Manual Humididty Reached" {
                  selector: "Manual Humididty Reached" -> [_ w1136]
                  frame False {
                  }
                  frame True {
                    n1215 = Not(x=w1136) -> (.not. x?=w1135:bool)
                    n1216 = local write "Manual Humididty Reached"(w1135) -> ()
                    n1217 = local read "EVENT LOG"() -> (w1138:string)
                    n1218 = call "Event Log.vi"("Content"="Target Humidity reached", "EVENT LOG"=w1138) -> ("EVENT LOG"=w1137:string)  [unwired: 8 in, 1 out]
                    n1219 = local write "EVENT LOG"(w1137) -> ()
                  }
                }
              }
            }
          }
        }
      }
      frame True {
        n1220 = local write "Manual Humididty Reached"(TRUE ("Manual Humididty Reached")) -> ()
      }
    }
    n1221 = local read "Cap Live Image"() -> (w1119:bool)
    n1222 = local read "SCAR MEASURMENT"() -> (w1122:enum32{"Auto Scar", "Manual Scar"})
    n1223 = Equal?(x=w1122, y=enum32{"Auto Scar", "Manual Scar"}."Manual Scar" ("SCAR MEASURMENT")) -> (x = y?=w1120:bool)
    n1224 = And(x=w1120, y=w1119) -> (x .and. y?=w1118:bool)
    n1225 = Wait (ms)(milliseconds to wait=u32 250) -> ()  [unwired: 1 out]
    n1226 = case shown="True" w1118 {
      selector: w1118 -> [_ w1441]
      frame False {
      }
      frame True {
        n1227 = stacked-sequence {
          tunnel: [_ _ _ w1460 _] -> _
          tunnel: w1441 -> [_ _ _ _ w1467]
          frame #0 {
            w1442 = 0.0
            n1228 = local write "Major Axis"(w1442) -> ()
            n1229 = local write "Minor Axis"(w1442) -> ()
            n1230 = local write "Average"(w1442) -> ()
          }
          frame #1 {
            n1231 = call "CAMERA LIVE FEED FGV.vi"("Enum - Menu"=CAMERA_LIVE_FEED_ENUM."CAMERA MINIMIZE") -> ()  [unwired: 9 in, 2 out]
          }
          frame #2 {
            n1232 = local read "Magnification len live scar"() -> (w1446:string)
            n1233 = case shown="\"10x\", Default" w1446 {
              tunnel: ["_10x" "_5x"] -> w1445
              frame "10x", Default {
              }
              frame "5x" {
              }
            }
            n1234 = local read "FILE 3"() -> (w1452:string)
            n1235 = call <vilib>:"Trim Whitespace.vi"("string"="C:\\LAB-IQ\\images\\") -> ("trimmed string"=w1454:string)  [unwired: 1 in]
            n1236 = String To Path(string=w1454) -> (path=w1453:path)
            n1237 = Concatenate Strings(w1452, w1445, ".png" ("string")) -> (w1451:string)
            n1238 = Build Path(base path=w1453, name or relative path=w1451) -> (appended path=w1450:path)
            n1239 = Path To String(path=w1450) -> (string=w1449:string)
            n1240 = call "CAMERA LIVE FEED FGV.vi"("Enum - Menu"=CAMERA_LIVE_FEED_ENUM."CAMERA SAVE", "Image Path"=w1449) -> ("error out"=w1447:errorcluster)  [unwired: 8 in, 1 out]
            n1241 = case shown="No Error" w1447 {
              frame No Error {
                n1242 = One Button Dialog(message="Image saved successfully") -> ()  [unwired: 1 in, 1 out]
              }
              frame Error {
              }
            }
          }
          frame #3 {
            n1243 = call "LIST FILE NAMES.vi"() -> ("error out"=w1462:errorcluster, "filenames"=w1459:string[])  [unwired: 10 in]
            n1244 = call "IMAGE ANALYSIS.vi"("Enum"=POST_ANALYSIS_ENUM."SHOW UI", "error in"=w1462) -> ("error out"=w1460:errorcluster)  [unwired: 8 in, 1 out]
            n1245 = property on="Test File List :" class="CmbBox"("Strings[]"=w1459) -> ()  [unwired: 2 in, 2 out]
          }
          frame #4 {
            (unwired) T26."Report" ("Main Dashboard Buttons")
            (unwired) T28."Report" ("Main Dashboard Buttons")
            n1246 = Not(x=w1467) -> (.not. x?=w1466:bool)
            n1247 = local write "Zoom Factore"(0.0 ("Zoom Factore")) -> ()
            n1248 = local write "Cap Live Image"(w1466) -> ()
            n1249 = local write "Main Tab"(T4."Adv Scar Report" ("Main Tab")) -> ()
            n1250 = property on="Cap Live Image" class="Bool (strict)"("BoolText.Text"="Capture Image" ("Boolean Text.Text")) -> ()  [unwired: 2 in, 2 out]
            n1251 = local write "Main Dashboard Buttons"(T1."Report" ("Main Dashboard Buttons")) -> ()
          }
        }
      }
    }
    n1252 = local read "change Gain"() -> (w1102:bool)
    n1253 = local read "Back Square"() -> (w1101:bool)
    n1254 = case shown="True" w1102 {
      selector: w1102 -> [_ w1146]
      frame False {
      }
      frame True {
        n1255 = stacked-sequence {
          tunnel: w1146 -> [_ w1154]
          frame #0 {
            n1256 = local read "Actual (µm)"() -> (w1150:dbl)
            n1257 = local read "Pixel Value"() -> (w1149:dbl)
            n1258 = local read "Magnification :"() -> (w1148:string)
            n1259 = Divide(x=w1150, y=w1149) -> (x/y=w1147:dbl)
            n1260 = case shown="\"10x\"" w1148 {
              tunnel: w1147 -> [w1151 w1152]
              frame "10x" {
                n1261 = local write "10x Gain"(w1151) -> ()
              }
              frame "5x", Default {
                n1262 = local write "5x Gain"(w1152) -> ()
              }
            }
          }
          frame #1 {
            n1263 = Not(x=w1154) -> (.not. x?=w1153:bool)
            n1264 = local write "change Gain"(w1153) -> ()
          }
        }
      }
    }
    n1265 = case shown="True" w1101 {
      selector: w1101 -> [_ w1144]
      frame False {
      }
      frame True {
        n1266 = Not(x=w1144) -> (.not. x?=w1143:bool)
        n1267 = local write "Back Square"(w1143) -> ()
        n1268 = local write "Calibration Tab"(enum32{"Measrument", "Calibrate"}."Measrument" ("Calibration Tab")) -> ()
      }
    }
    n1269 = local read "Rectangle Tool"() -> (w1113:bool)
    n1270 = local read "Clear ROI Tool"() -> (w1112:bool)
    n1271 = local read "Open Image"() -> (w1117:bool)
    n1272 = local read "line tool"() -> (w1114:bool)
    n1273 = local read "OUT"() -> (w1115:bool)
    n1274 = local read "In"() -> (w1116:bool)
    n1275 = case shown="True" w1117 {
      selector: w1117 -> [_ w1427]
      tunnel: [w1418 w1429] -> _
      tunnel: w1107 -> [w1418 w1428]
      frame False {
      }
      frame True {
        w1422 = "_5x" ("regular expression")
        n1276 = Not(x=w1427) -> (.not. x?=w1426:bool)
        n1277 = local write "Open Image"(w1426) -> ()
        n1278 = call "IMAGE ANALYSIS.vi"("Enum"=POST_ANALYSIS_ENUM."HIDE UI", "error in"=w1428) -> ("error out"=w1436:errorcluster)  [unwired: 8 in, 1 out]
        n1279 = call <vilib>:"Clear Errors.vi"("error in (no error)"=w1436) -> ("error out"=w1419:errorcluster)  [unwired: 5 in, 1 out]
        n1280 = call "File Dialog"("start path"=path "C:/LAB-IQ/images", "error in"=w1419) -> ("selected path"=w1421:path, "error out"=w1434:errorcluster)  [unwired: 10 in, 2 out]
        "Image path  2" <- w1421
        n1281 = call <vilib>:"Clear Errors.vi"("error in (no error)"=w1434) -> ("error out"=w1433:errorcluster)  [unwired: 5 in, 1 out]
        n1282 = call "IMAGE ANALYSIS.vi"("Enum"=POST_ANALYSIS_ENUM."OPEN FILE", "error in"=w1433, "File Path"=w1421) -> ("error out"=w1432:errorcluster)  [unwired: 7 in, 1 out]
        n1283 = call <vilib>:"Clear Errors.vi"("error in (no error)"=w1432) -> ("error out"=w1431:errorcluster)  [unwired: 5 in, 1 out]
        n1284 = call "IMAGE ANALYSIS.vi"("Enum"=POST_ANALYSIS_ENUM."SHOW UI", "error in"=w1431) -> ("error out"=w1429:errorcluster)  [unwired: 8 in, 1 out]
